vi "HEWH General Start End Draw.vi"(8 "error in (no error)":errorcluster, 10 "Full Data Input":string[][](array[string]), 11 "Start Index":i32) -> (0 "error out":errorcluster, 3 "End Index":i32)   [LabVIEW 2016]
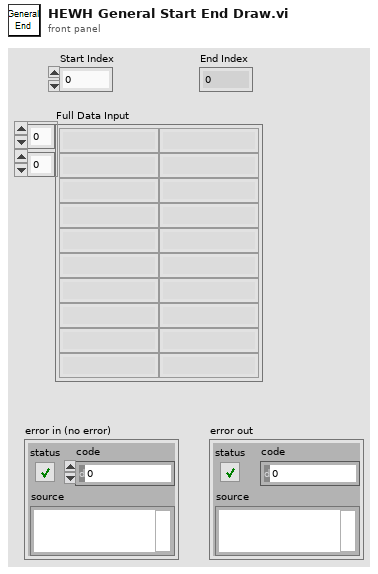
[diagram p1: front panel]
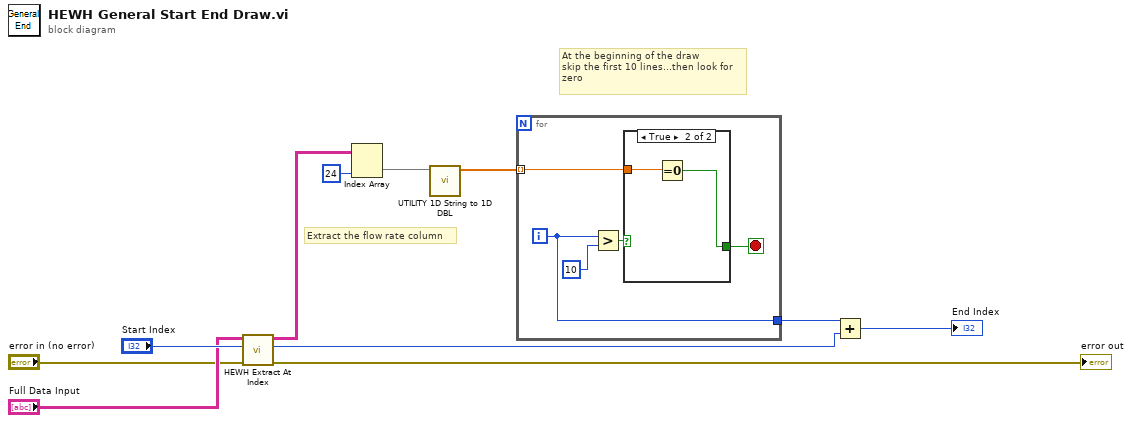
[diagram p0: block diagram]
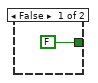
[diagram p2: hidden frame]
diagram:
  # "Extract the flow rate column"
  # "At the beginning of the draw\nskip the first 10 lines...then look for\nzero"
  n1 = call "HEWH Extract At Index.vi"("Error In"="error in (no error)", "Test Start Index in"="Start Index", "all rows in"="Full Data Input") -> ("Error Out"=→"error out":errorcluster, "Test Start Index out"=w6:i32, "Array"=w3:string[][])  [unwired: 6 in]
  n2 = Index Array(array=w3, index (col)=24 ("disabled index (col)")) -> (element=w1:string[])  [unwired: 1 in]
  n3 = call "UTILITY 1D String to 1D DBL.vi"("Save Data"=w1) -> ("DBL"=w4:dbl[])  [unwired: 10 in]
  n4 = for {
    tunnel: w4 -> [w13] mode=indexing
    tunnel: [w12] -> w5
    i -> [w12]
    stop <- w14 stop-if-true
    n5 = Greater?(x=w12, y=10) -> (0:w15:bool)
    n6 = case shown="True" w15 {
      tunnel: [FALSE w18] -> w14
      tunnel: w13 -> [_ w19]
      frame False {
      }
      frame True {
        n7 = Equal To 0?(x=w19) -> (x = 0?=w18:bool)
      }
    }
  }
  n8 = Add(x=w5, y=w6) -> (x+y=→"End Index":i32)
